vi "HostExampleWith8AuxDio.vi"() -> ()   [LabVIEW 2023]
uses:
  github26-test/flexrio-custom/deps/hdl-shared/host_interfaces/fifo/LabVIEW/HdlFifo/NiFpga_HdlFifo_WriteI32.vi
  github26-test/flexrio-custom/deps/hdl-shared/host_interfaces/fifo/LabVIEW/HdlFifo/NiFpga_HdlFifo_ReadI32.vi
  <vilib>/FPGAPlugInAG/Dynamic/niLvFpga_Download_Dynamic.vi
  <vilib>/FPGAPlugInAG/Dynamic/niLvFpga_Run_Dynamic.vi
  github26-test/flexrio-custom/deps/hdl-shared/host_interfaces/fifo/LabVIEW/HdlFifo/NiFpga_HdlFifo_AddI32.vi
  github26-test/flexrio-custom/deps/hdl-shared/host_interfaces/fifo/LabVIEW/HdlFifo/private/_NiFpga_HdlFifo_GetStream.vi
  <vilib>/Utility/error.llb/Error Cluster From Error Code.vi
  <vilib>/rvi/interface/nirviMethod/nirviMethod.xnode
panel:
  in  "Read Dig In and Status":bool
  out "Digital Input and Status":u32 format="%.0x"
  in  "Write Dig Direction":bool
  in  "Digital Direction":u32 format="%.0x"
  in  "Write Dig Out Data":bool
  in  "Digital Output Data":u32 format="%.0x"
  in  "Device address":string
  in  "Bitfile path":path
  out "empty elements remaining":u64
  out "Elements Remaining":u64
  out "error out":errorcluster
  in  "WriteScratch":bool
  in  "ReadScratch":bool
  out "Scratch Read":u32 format="%.0x"
  in  "Scratch Write":u32 format="%.0x"
  in  "Num Elements":i32
  out "Read Data":u32[](array[numeric])
  in  "Read FPGA FIFO":bool
  in  "Write FPGA FIFO":bool
  in  "Write Data":u32[](array[numeric])
  in  "WriteReg":bool
  in  "ReadReg":bool
  out "Read Value":u32 format="%.0x"
  in  "Write Value":u32 format="%.0x"
  in  "Write Offset":u32 format="%.0x"
  in  "Read Offset":u32 format="%.0x"
  in  "Num Elements":i32
  out "Data 4":i32[](array[numeric])
  in  "Write Data":i32[](array[numeric])
  in  "Read Host FIFO":bool
  in  "Write Host FIFO":bool
  out "Numeric":i32
  in  "stop":bool
  # "Write and read any register offset"
  # "Write and read the scratch register"
  # "Scratch Register"
  # "Write and read the Host to FPGA FIFO"
  # "Host to FPGA FIFO"
  # "Write and Read Digital Lines"
  # "[0:7] - Digital Input Data\n[8:15] - Done Status"
  # "Write and read the FPGA to Host FIFO"
  # "FPGA to Host FIFO"
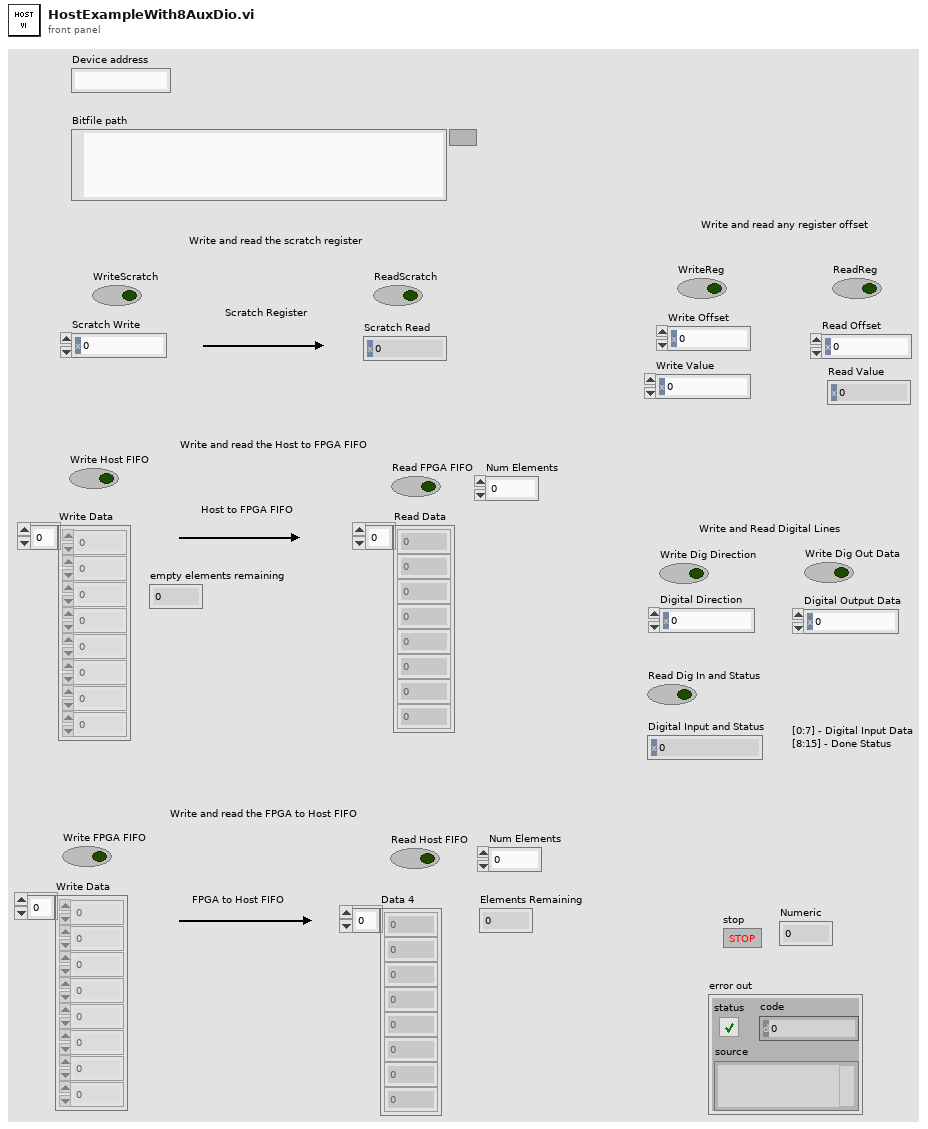
[diagram p1: front panel]
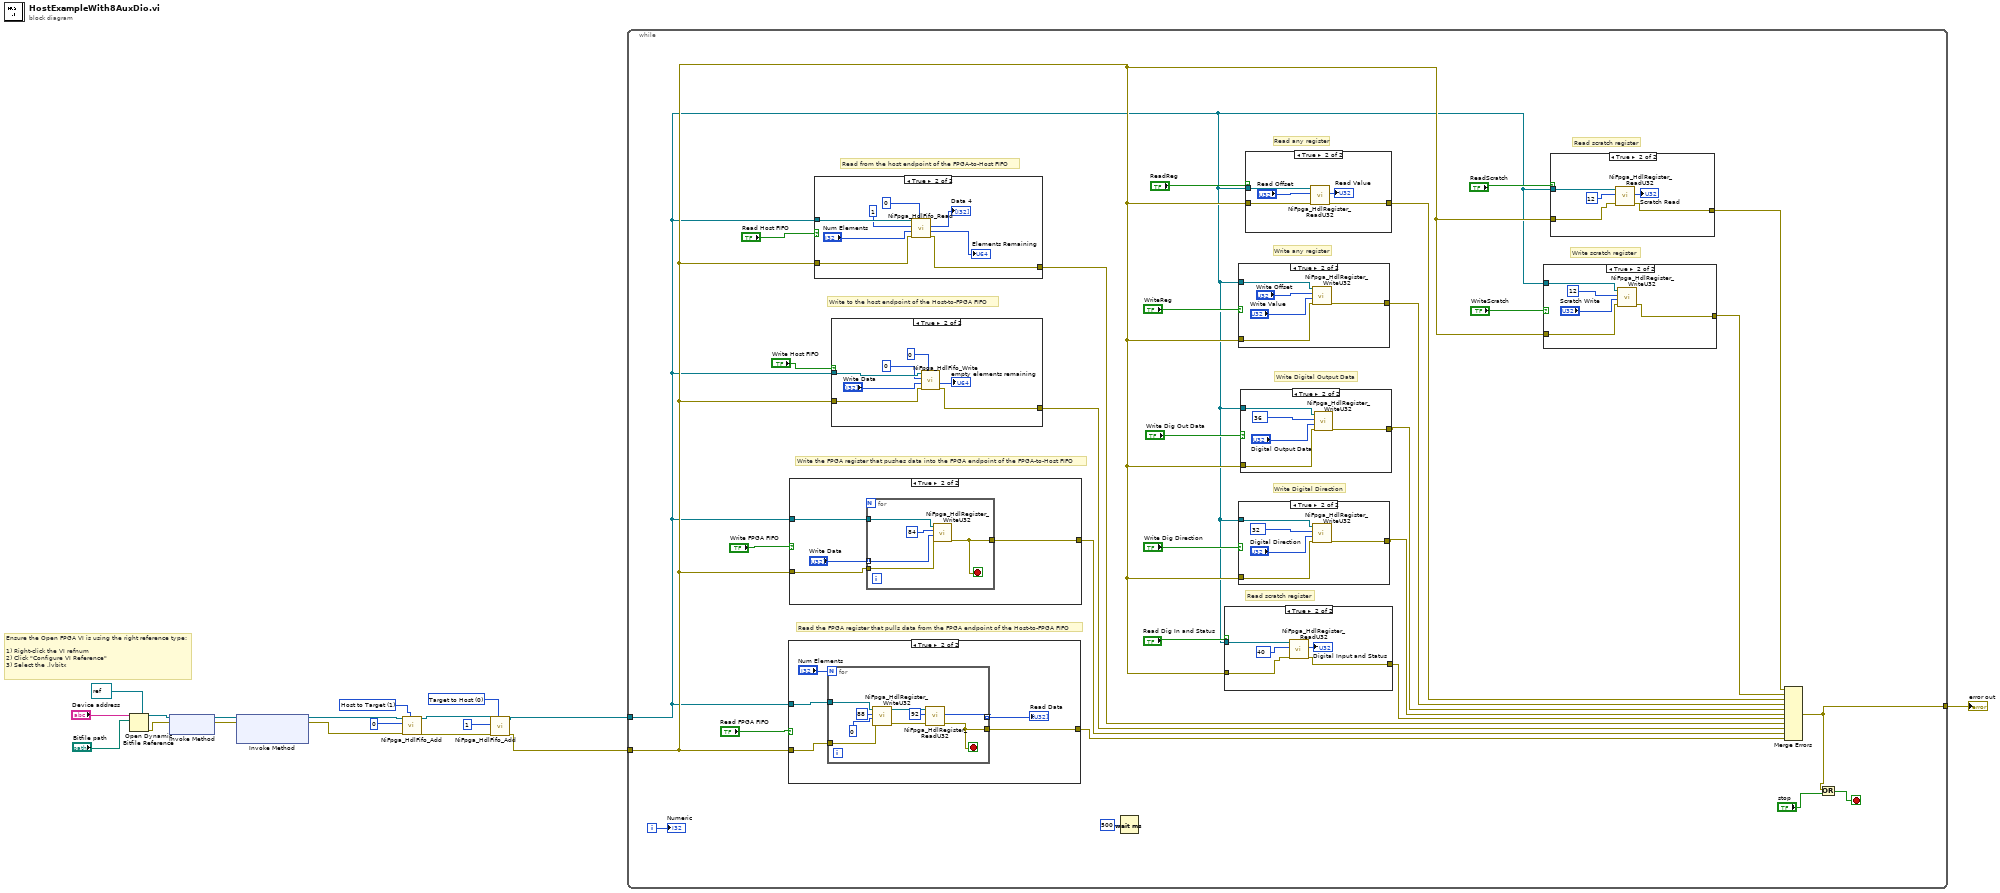
[diagram p0: block diagram]
diagram:
  w4 = u32 0 items=["Target to Host", "Host to Target"] ("direction")
  w10 = u32 1 items=["Target to Host", "Host to Target"]
  # "Ensure the Open FPGA VI is using the right reference type:\n\n1) Right-click the VI refnum \n2) Click \"Configure VI Reference\"\n3) Select the .lvbitx"
  n1 = Open Dynamic Bitfile Reference(0:"Device address", 1:"Bitfile path", 4:refnum<k20> refnum ("Type")) -> (5:w15:refnum<k20>, 8:w14:errorcluster)  [unwired: 2 in]
  n2 = xnode "Invoke Method"("FPGA VI Reference In"=w15, "error in"=w14) -> ("FPGA VI Reference Out"=w17:refnum<k20>, "error out"=w18:errorcluster)
  n3 = xnode "Invoke Method"("FPGA VI Reference In"=w17, "error in"=w18) -> ("FPGA VI Reference Out"=w11:refnum<k20>, "error out"=w5:errorcluster)  [unwired: 1 in]
  n4 = call-poly "NiFpga_HdlFifo_Add.vi"("direction"=w10, "error in (no error)"=w5, "Fifo Number"=u32 0, "FPGA VI Reference In"=w11) -> ("error out"=w3:errorcluster, "FPGA VI Reference Out"=w7:refnum<k20>)  [unwired: 6 in]
  n5 = call-poly "NiFpga_HdlFifo_Add.vi"("direction"=w4, "error in (no error)"=w3, "Fifo Number"=u32 1, "FPGA VI Reference In"=w7) -> ("error out"=w2:errorcluster, "FPGA VI Reference Out"=w8:refnum<k20>)  [unwired: 6 in]
  n6 = while {
    tunnel: w8 -> [w22]
    tunnel: w2 -> [w23]
    tunnel: [w27] -> w1
    i -> [w47]
    stop <- w29 stop-if-true
    # "Read scratch register"
    # "Write Digital Direction"
    # "Write Digital Output Data"
    # "Write scratch register"
    # "Read scratch register"
    # "Read any register"
    # "Write any register"
    # "Read from the host endpoint of the FPGA-to-Host FIFO"
    # "Write to the host endpoint of the Host-to-FPGA FIFO"
    # "Read the FPGA register that pulls data from the FPGA endpoint of the Host-to-FPGA FIFO"
    # "Write the FPGA register that pushes data into the FPGA endpoint of the FPGA-to-Host FIFO"
    n7 = case shown="True" "Read FPGA FIFO" {
      tunnel: w22 -> [_ w83]
      tunnel: w23 -> [w78 w80]
      tunnel: [w78 w79] -> w30
      frame False {
      }
      frame True {
        n8 = for {
          N: "Num Elements" -> [_]
          tunnel: w83 -> [w92]
          tunnel: [w88] -> w82 mode=indexing
          tunnel: w80 -> [w86]
          tunnel: [w84] -> w79
          stop <- w84 stop-if-true
          n9 = call "NiFpga_HdlRegister_WriteU32.vi"("error in (no error)"=w86, "Value"=u32 0, "Offset"=u32 88, "FPGA VI Reference In"=w92) -> ("error out"=w85:errorcluster, "FPGA VI Reference Out"=w90:refnum<k20>)  [unwired: 5 in]
          n10 = call "NiFpga_HdlRegister_ReadU32.vi"("error in (no error)"=w85, "Offset"=u32 92, "FPGA VI Reference In"=w90) -> ("error out"=w84:errorcluster, "Value"=w88:u32)  [unwired: 6 in, 1 out]
        }
        "Read Data" <- w82
      }
    }
    n11 = case shown="True" "Write FPGA FIFO" {
      tunnel: w22 -> [_ w97]
      tunnel: w23 -> [w93 w95]
      tunnel: [w93 w94] -> w31
      frame False {
      }
      frame True {
        n12 = for {
          tunnel: w97 -> [w102]
          tunnel: "Write Data" -> [w100] mode=indexing
          tunnel: w95 -> [w99]
          tunnel: [w98] -> w94
          stop <- w98 stop-if-true
          n13 = call "NiFpga_HdlRegister_WriteU32.vi"("error in (no error)"=w99, "Value"=w100, "Offset"=u32 84, "FPGA VI Reference In"=w102) -> ("error out"=w98:errorcluster)  [unwired: 5 in, 1 out]
        }
      }
    }
    n14 = case shown="True" "Read Host FIFO" {
      tunnel: w22 -> [_ w130]
      tunnel: w23 -> [w123 w125]
      tunnel: [w123 w124] -> w33
      frame False {
      }
      frame True {
        n15 = call-poly "NiFpga_HdlFifo_Read.vi"("timeout"=u32 0, "error in (no error)"=w125, "number of elements"="Num Elements", "fifo number"=u32 1 ("Fifo Number"), "fpga vi reference in"=w130) -> ("error out"=w124:errorcluster, "elements remaining"=→"Elements Remaining":u64, "data out"=→"Data 4":i32[])  [unwired: 2 in, 1 out]
      }
    }
    n16 = case shown="True" "Write Host FIFO" {
      tunnel: w22 -> [_ w121]
      tunnel: w23 -> [w115 w117]
      tunnel: [w115 w116] -> w32
      frame False {
      }
      frame True {
        n17 = call-poly "NiFpga_HdlFifo_Write.vi"("timeout"=u32 0, "error in (no error)"=w117, "data in"="Write Data", "fifo number"=u32 0 ("Fifo Number 2"), "fpga vi reference in"=w121) -> ("error out"=w116:errorcluster, "empty elements remaining"=→"empty elements remaining":u64)  [unwired: 3 in, 1 out]
      }
    }
    n18 = Wait (ms)(milliseconds to wait=u32 500) -> ()  [unwired: 1 out]
    n19 = case shown="True" "Read Dig In and Status" {
      tunnel: w22 -> [_ w53]
      tunnel: w23 -> [w48 w50]
      tunnel: [w48 w49] -> w19
      frame False {
      }
      frame True {
        n20 = call "NiFpga_HdlRegister_ReadU32.vi"("error in (no error)"=w50, "Offset"=u32 40 ("Read Offset 2"), "FPGA VI Reference In"=w53) -> ("error out"=w49:errorcluster, "Value"=→"Digital Input and Status":u32)  [unwired: 6 in, 1 out]
      }
    }
    n21 = case shown="True" "WriteReg" {
      tunnel: w22 -> [_ w108]
      tunnel: w23 -> [w103 w105]
      tunnel: [w103 w104] -> w34
      frame False {
      }
      frame True {
        n22 = call "NiFpga_HdlRegister_WriteU32.vi"("error in (no error)"=w105, "Value"="Write Value", "Offset"="Write Offset", "FPGA VI Reference In"=w108) -> ("error out"=w104:errorcluster)  [unwired: 5 in, 1 out]
      }
    }
    n23 = case shown="True" "Write Dig Direction" {
      tunnel: w22 -> [_ w59]
      tunnel: w23 -> [w54 w56]
      tunnel: [w54 w55] -> w20
      frame False {
      }
      frame True {
        n24 = call "NiFpga_HdlRegister_WriteU32.vi"("error in (no error)"=w56, "Value"="Digital Direction", "Offset"=u32 32 ("Write Offset 2"), "FPGA VI Reference In"=w59) -> ("error out"=w55:errorcluster)  [unwired: 5 in, 1 out]
      }
    }
    n25 = case shown="True" "Write Dig Out Data" {
      tunnel: w22 -> [_ w65]
      tunnel: w23 -> [w60 w62]
      tunnel: [w60 w61] -> w21
      frame False {
      }
      frame True {
        n26 = call "NiFpga_HdlRegister_WriteU32.vi"("error in (no error)"=w62, "Value"="Digital Output Data", "Offset"=u32 36 ("Write Offset 2"), "FPGA VI Reference In"=w65) -> ("error out"=w61:errorcluster)  [unwired: 5 in, 1 out]
      }
    }
    n27 = case shown="True" "ReadReg" {
      tunnel: w22 -> [_ w114]
      tunnel: w23 -> [w109 w111]
      tunnel: [w109 w110] -> w35
      frame False {
      }
      frame True {
        n28 = call "NiFpga_HdlRegister_ReadU32.vi"("error in (no error)"=w111, "Offset"="Read Offset", "FPGA VI Reference In"=w114) -> ("error out"=w110:errorcluster, "Value"=→"Read Value":u32)  [unwired: 6 in, 1 out]
      }
    }
    n29 = case shown="True" "WriteScratch" {
      tunnel: w22 -> [_ w71]
      tunnel: w23 -> [w66 w68]
      tunnel: [w66 w67] -> w36
      frame False {
      }
      frame True {
        n30 = call "NiFpga_HdlRegister_WriteU32.vi"("error in (no error)"=w68, "Value"="Scratch Write", "Offset"=u32 12 ("Write Offset 2"), "FPGA VI Reference In"=w71) -> ("error out"=w67:errorcluster)  [unwired: 5 in, 1 out]
      }
    }
    n31 = case shown="True" "ReadScratch" {
      tunnel: w22 -> [_ w77]
      tunnel: w23 -> [w72 w74]
      tunnel: [w72 w73] -> w37
      frame False {
      }
      frame True {
        n32 = call "NiFpga_HdlRegister_ReadU32.vi"("error in (no error)"=w74, "Offset"=u32 12 ("Read Offset 2"), "FPGA VI Reference In"=w77) -> ("error out"=w73:errorcluster, "Value"=→"Scratch Read":u32)  [unwired: 6 in, 1 out]
      }
    }
    n33 = Merge Errors(w37, w36, w35, w34, w21, w20, w19, w33, w32, w31, w30) -> (w27:errorcluster)
    n34 = Or(x=w27, y="stop") -> (x .or. y?=w29:bool)
    "Numeric" <- w47
  }
  "error out" <- w1
